vi "VESASignal_Output.vi"(1 "h_Pixel":i16, 4 "v_Pixel":i16) -> ()   [LabVIEW 2018]
uses:
  <vilib>/rvi/Emulation/niFpgaEmulationIsFPGAContextNoSignature.vi
  <vilib>/rvi/Emulation/niFpgaSctlEmulationGetInTimedLoop.vi
  <vilib>/rvi/errors/niFpgaSetErrorForExecOnDevCompSimple.vi
  <vilib>/rvi/eio/common/nirviEmuReportErrorAndStop.vi
  <vilib>/rvi/DataTransferAndStorage/Container/Common/niFpgaContainerGetUniqueNameForEmu.vi
  <vilib>/rvi/FIFO/Fifo_Resource/nirvififoEmulationSetSize.vi
  <vilib>/rvi/FIFO/Fifo_Resource/nirviFifoEmulationQueueMgr.vi
  <instcachedir>/0/nirviFifoEmulationQueueMgr_E5CAEC123FF24DC58D834DCA3CDAA9B5.lvgen/nirviFifoEmulationQueueMgr_E5CAEC123FF24DC58D834DCA3CDAA9B5_002.vi
  <vilib>/Utility/error.llb/Clear Errors.vi
  <vilib>/rvi/FIFO/Fifo_Resource/nirvififoEmulationCreateLock.vi
  <vilib>/rvi/Emulation/niFpgaProcessEmulError.vi
  <vilib>/rvi/FIFO/Fifo_Resource/nirvififoEmulationObtainLock.vi
  <vilib>/rvi/FIFO/Fifo_Resource/nirvififoEmulationReleaseLock.vi
  <vilib>/rvi/occurrence/nirviWaitOnOccurrenceBase.vi
  <vilib>/rvi/errors/nirviReportUnexpectedCaseInternalError.vi
  <vilib>/rvi/errors/nirviReportUnexpectedCaseInternalError (U32).vi
  <vilib>/rvi/eio/common/nirviEmuTemplateMethod_errors.vi
  <vilib>/rvi/DataTransferAndStorage/Container/XNode/niFpgaContainer.xnode
  <vilib>/rvi/FIFO/Fifo_Resource/nirvififoEmulationRead.vi
  <vilib>/eio/EIONode/EIONode.xnode
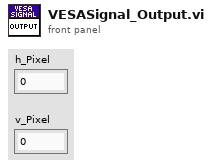
[diagram p1: front panel]
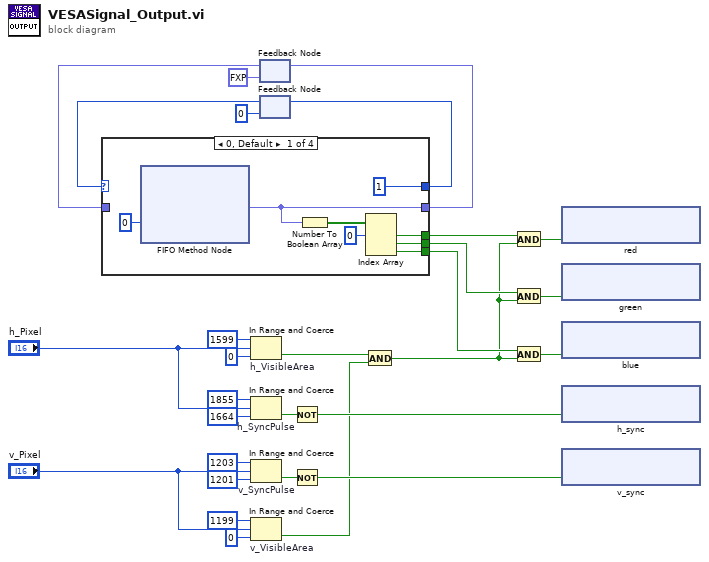
[diagram p0: block diagram]
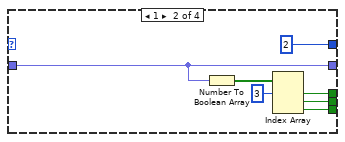
[diagram p2: hidden frame]
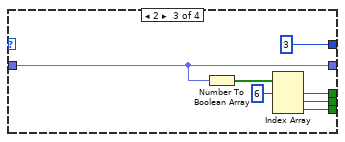
[diagram p3: hidden frame]
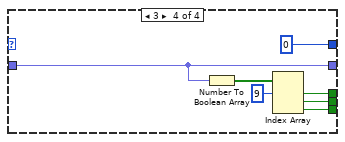
[diagram p4: hidden frame]
diagram:
  n1 = In Range and Coerce "h_VisibleArea"(upper limit=i16 1599, x="h_Pixel", lower limit=i16 0) -> (In Range?=w17:bool)  [unwired: 1 out]
  n2 = In Range and Coerce "h_SyncPulse"(upper limit=i16 1855, x="h_Pixel", lower limit=i16 1664) -> (In Range?=w26:bool)  [unwired: 1 out]
  n3 = In Range and Coerce "v_SyncPulse"(upper limit=i16 1203, x="v_Pixel", lower limit=i16 1201) -> (In Range?=w29:bool)  [unwired: 1 out]
  n4 = In Range and Coerce "v_VisibleArea"(upper limit=i16 1199, x="v_Pixel", lower limit=i16 0) -> (In Range?=w16:bool)  [unwired: 1 out]
  n5 = feedback #1(fxp<+,12,12> 0.0 ("Element")) -> (w10:fxp<+,12,12>)
  n6 = feedback #2(i8 0) -> (w11:i8)
  n7 = case shown="0, Default" w11 {
    tunnel: [i8 1 i8 2 i8 3 i8 0] -> w12
    tunnel: [w30 w38 w45 w52] -> w9
    tunnel: w10 -> [_ w38 w45 w52]
    tunnel: [w33 w41 w48 w55] -> w8
    tunnel: [w32 w40 w47 w54] -> w7
    tunnel: [w31 w39 w46 w53] -> w6
    frame 0, Default {
      n8 = xnode ("FIFO Method Node")("Timeout"=0) -> ("Element"=w30:fxp<+,12,12>)  [unwired: 1 in, 2 out]
      n9 = Number To Boolean Array(number=w30) -> (Boolean array=w35:bool[])
      n10 = Index Array(array=w35, index #1=0 ("index")) -> (element #1=w33:bool, element #2=w32:bool, element #3=w31:bool)  [unwired: 2 in]
    }
    frame 1 {
      n11 = Number To Boolean Array(number=w38) -> (Boolean array=w43:bool[])
      n12 = Index Array(array=w43, index #1=3 ("index")) -> (element #1=w41:bool, element #2=w40:bool, element #3=w39:bool)  [unwired: 2 in]
    }
    frame 2 {
      n13 = Number To Boolean Array(number=w45) -> (Boolean array=w50:bool[])
      n14 = Index Array(array=w50, index #1=6 ("index")) -> (element #1=w48:bool, element #2=w47:bool, element #3=w46:bool)  [unwired: 2 in]
    }
    frame 3 {
      n15 = Number To Boolean Array(number=w52) -> (Boolean array=w57:bool[])
      n16 = Index Array(array=w57, index #1=9 ("index")) -> (element #1=w55:bool, element #2=w54:bool, element #3=w53:bool)  [unwired: 2 in]
    }
  }
  n17 = feedback-in #1(w9) -> ()
  n18 = feedback-in #2(w12) -> ()
  n19 = Not(x=w26) -> (.not. x?=w23:bool)
  n20 = Not(x=w29) -> (.not. x?=w22:bool)
  n21 = And(x=w17, y=w16) -> (x .and. y?=w1:bool)
  n22 = And(x=w8, y=w1) -> (x .and. y?=w15:bool)
  n23 = And(x=w7, y=w1) -> (x .and. y?=w14:bool)
  n24 = And(x=w6, y=w1) -> (x .and. y?=w13:bool)
  n25 = xnode "red"("ConnectorC/DIO0"=w15) -> ()  [unwired: 1 in, 1 out]
  n26 = xnode "green"("ConnectorC/DIO1"=w14) -> ()  [unwired: 1 in, 1 out]
  n27 = xnode "blue"("ConnectorC/DIO2"=w13) -> ()  [unwired: 1 in, 1 out]
  n28 = xnode "h_sync"("ConnectorC/DIO3"=w23) -> ()  [unwired: 1 in, 1 out]
  n29 = xnode "v_sync"("ConnectorC/DIO4"=w22) -> ()  [unwired: 1 in, 1 out]
